vi "to string.vi"(8 "error in":errorcluster, 11 "tag bus configurable plugin module configuration in":refnum<class "tag bus configurable plugin module configuration.lvclass">) -> (0 "error out":errorcluster, 1 "data":string, 2 "version":string, 3 "tag bus configurable plugin module configuration out":refnum<class "tag bus configurable plugin module configuration.lvclass">)   [LabVIEW 2013, in "tag bus configurable plugin module configuration.lvclass"]
doc: "Provides an interface for saving a module configuration to a file or other serialized data source. It is recommended that all children of this class store data in two sets--data required for its own initialization, and any data required for parent initialization--and that each implementation uses the <b>Call Parent Method</b> primitive to serialize parent information."
uses:
  tag bus configurable plugin module configuration.lvclass
  <vilib>/NI/Tag Bus Module Framework/module configuration/TBM module configuration.lvclass
  tag bus configurable plugin module configuration.lvclass/tag bus configurable plugin module configuration.ctl
  current version.vi
  <vilib>/NI/Configuration Framework/serializable configuration/NISE_CEF_serializable configuration.lvclass
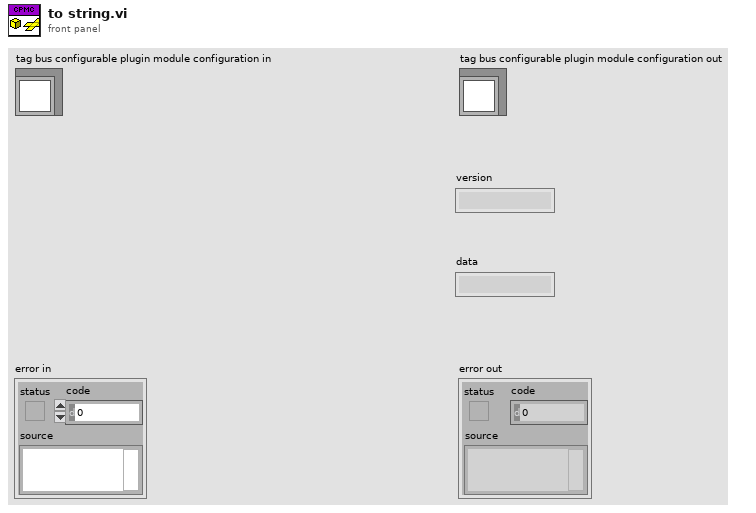
[diagram p1: front panel]
types:
  T1 = typedef "tag bus configurable plugin module configuration.lvclass/Line.ctl" = cluster{"channel":refnum<class "TBM channel.lvclass">}
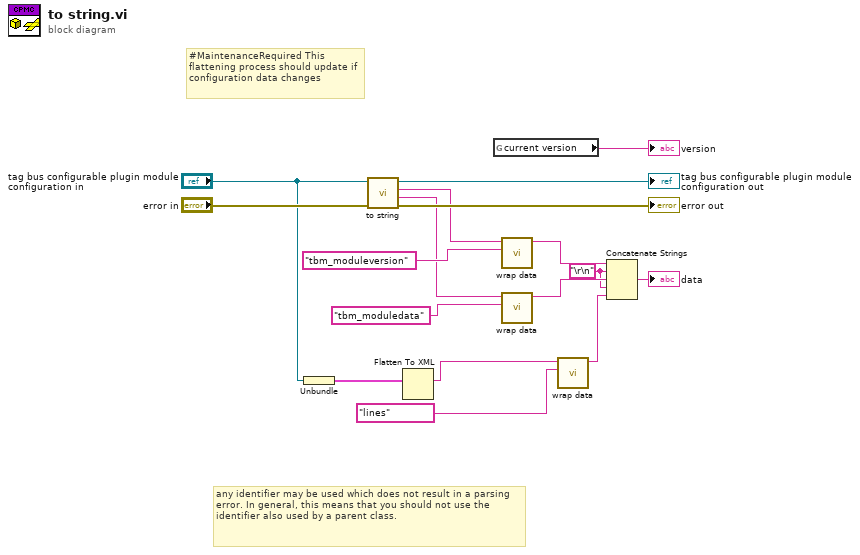
[diagram p0: block diagram]
diagram:
  w3 = "\r\n"
  # "any identifier may be used which does not result in a parsing error. In general, this means that you should not use the identifier also used by a parent class."
  # "#MaintenanceRequired This flattening process should update if configuration data changes"
  n1 = Unbundle("tag bus configurable plugin module configuration in") -> (w2:T1[])
  n2 = call-parent "to string.vi"("error in"="error in", "module configuration in"="tag bus configurable plugin module configuration in") -> ("error out"=→"error out":errorcluster, "data"=w8:string, "version"=w9:string, "module configuration out"=→"tag bus configurable plugin module configuration out":refnum<class "tag bus configurable plugin module configuration.lvclass">)  [unwired: 6 in]
  n3 = Flatten To XML(anything=w2) -> (xml string=w1:string)
  n4 = global read "current version.vi" "current version"() -> (→"version":string)
  n5 = call <vilib>:"wrap data.vi"("identifier"="tbm_moduleversion" ("additional identifier"), "data to wrap"=w9) -> ("wrapped data"=w11:string)  [unwired: 9 in]
  n6 = call <vilib>:"wrap data.vi"("identifier"="tbm_moduledata" ("additional identifier"), "data to wrap"=w8) -> ("wrapped data"=w10:string)  [unwired: 9 in]
  n7 = call <vilib>:"wrap data.vi"("identifier"="lines" ("additional identifier"), "data to wrap"=w1) -> ("wrapped data"=w5:string)  [unwired: 9 in]
  n8 = Concatenate Strings(w11, w3, w10, w3, w5) -> (→"data":string)
